vi "Get Multiplexer.vi"(8 "error in":errorcluster, 11 "SDO Transfer in":refnum<class "SDO Transfer.lvclass">) -> (0 "error out":errorcluster, 2 "Multiplexer":cluster{"Index":u16, "Sub-Index":u8} {"Sub-Index" format="%02x"; "Index" format="%04x"}, 3 "SDO Transfer out":refnum<class "SDO Transfer.lvclass">)   [LabVIEW 2020, in "SDO Manager.lvlib" / "SDO Transfer.lvclass"]
uses:
  SDO Transfer.lvclass
  SDO Transfer.lvclass/SDO Transfer.ctl
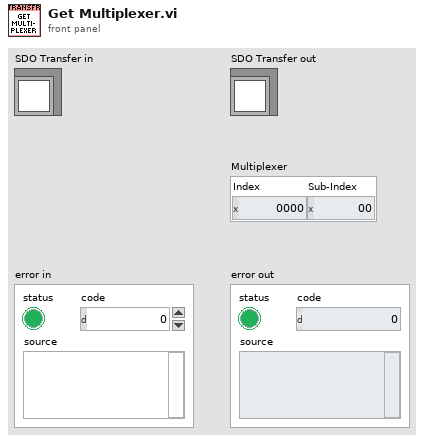
[diagram p1: front panel]
types:
  T1 = typedef "CANopen.lvlib/Multiplexer.ctl" = cluster{"Index":u16, "Sub Index":u8}
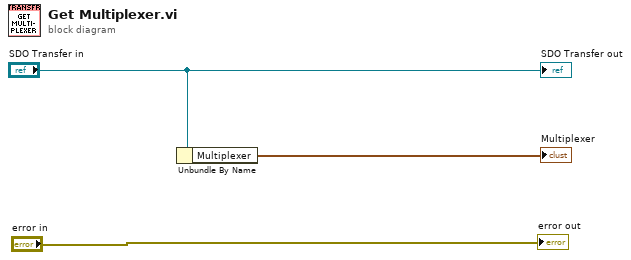
[diagram p0: block diagram]
diagram:
  n1 = Unbundle By Name("SDO Transfer in") -> ("Multiplexer"=→"Multiplexer":T1)
  "error out" <- "error in"
  "SDO Transfer out" <- "SDO Transfer in"
